vi "Get Key Value (String Array).vi"(5 "Key name":string, 6 "Default value":string[](array[string]), 7 "Section name":string, 8 "error in (no error)":errorcluster, 10 "Strip Whitespace? [T]":bool=TRUE, 11 "Carya Config in":refnum<class "Carya Config.lvclass">) -> (0 "error out":errorcluster, 1 "Found?":bool, 2 "value":string[](array[string]), 3 "Carya Config out":refnum<class "Carya Config.lvclass">)   [LabVIEW 2013, in "Carya Config.lvclass"]
doc: "Copyright 2018, Carya Automatisering, Wiebe Walstra."
uses:
  Carya Config.lvclass
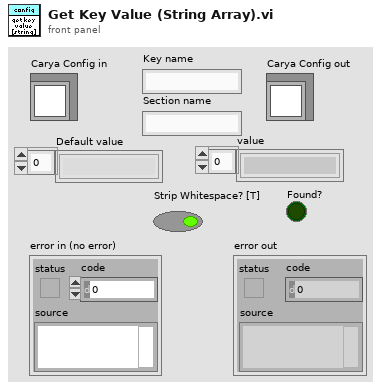
[diagram p1: front panel]
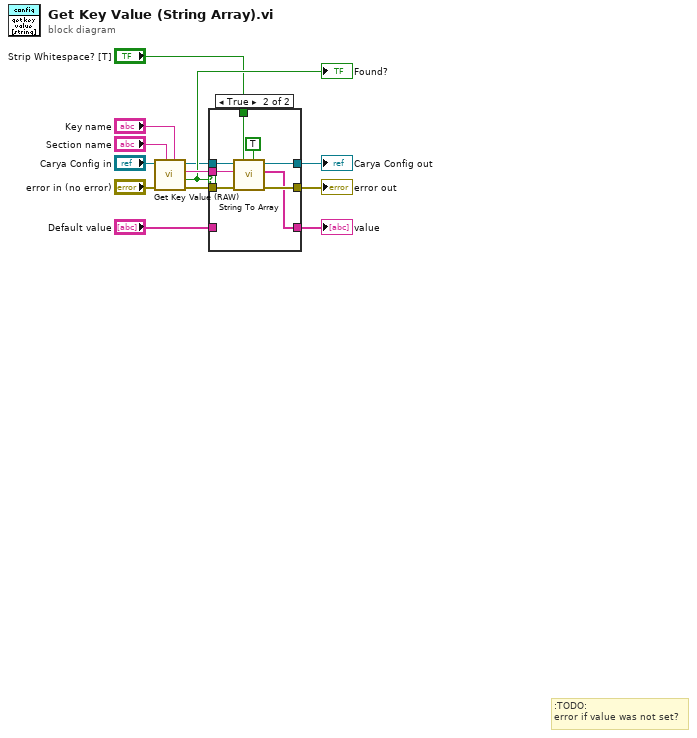
[diagram p0: block diagram]
diagram:
  # ":TODO:\nerror if value was not set?"
  n1 = call-dynamic "Get Key Value (RAW).vi"("Key name"="Key name", "Section name"="Section name", "error in (no error)"="error in (no error)", "Carya Config in"="Carya Config in") -> ("error out"=w12:errorcluster, "Found?"=w5:bool, "Value"=w7:string, "Carya Config out"=w3:refnum<class "Carya Config.lvclass">)  [unwired: 4 in]
  "Found?" <- w5
  n2 = case shown="True" w5 {
    tunnel: w12 -> [w15 w22]
    tunnel: [w15 w21] -> w8
    tunnel: w7 -> [_ w24]
    tunnel: "Default value" -> [w16 _]
    tunnel: [w16 w17] -> w4
    tunnel: w3 -> [w14 w23]
    tunnel: [w14 w20] -> w2
    tunnel: "Strip Whitespace? [T]" -> [_ w19]
    frame False {
    }
    frame True {
      n3 = call-dynamic "String To Array.vi"("Unescape? [F]"=TRUE, "Strip Whitespace? [T]"=w19, "error in (no error)"=w22, "resulting string"=w24, "Registry Object"=w23) -> ("error out"=w21:errorcluster, "Array"=w17:string[], "Registry Object"=w20:refnum<class "Carya Config.lvclass">)  [unwired: 4 in]
    }
  }
  "error out" <- w8
  "Carya Config out" <- w2
  "value" <- w4
